vi "inner_product.vi"(8 "L2ENDpos":cluster{"X":sgl, "Y":sgl}={"X"=7.0, "Y"=2.0}, 9 "L2STARTpos":cluster{"X":sgl, "Y":sgl}={"X"=2.0, "Y"=2.0}, 10 "L1ENDpos":cluster{"X":sgl, "Y":sgl}={"X"=1.0, "Y"=1.0}, 11 "L1STARTpos":cluster{"X":sgl, "Y":sgl}={"X"=0.0, "Y"=1.0}) -> (3 "数值":dbl format="%#_13g")   [LabVIEW 2018]
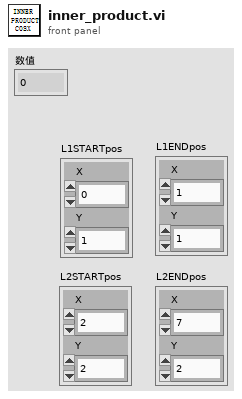
[diagram p1: front panel]
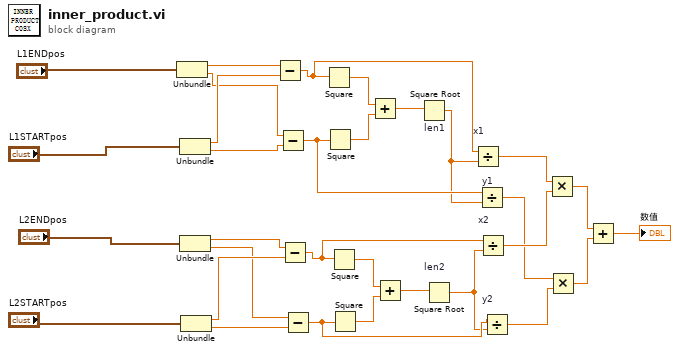
[diagram p0: block diagram]
diagram:
  n1 = Unbundle("L1ENDpos") -> ("X"=w27:sgl, "Y"=w25:sgl)
  n2 = Unbundle("L1STARTpos") -> ("X"=w26:sgl, "Y"=w24:sgl)
  n3 = Unbundle("L2ENDpos") -> ("X"=w17:sgl, "Y"=w15:sgl)
  n4 = Unbundle("L2STARTpos") -> ("X"=w16:sgl, "Y"=w14:sgl)
  n5 = Subtract(x=w27, y=w26) -> (x-y=w13:sgl)
  n6 = Subtract(x=w25, y=w24) -> (x-y=w11:sgl)
  n7 = Subtract(x=w17, y=w16) -> (x-y=w12:sgl)
  n8 = Subtract(x=w15, y=w14) -> (x-y=w9:sgl)
  n9 = Square(x=w13) -> (x^2=w23:sgl)
  n10 = Square(x=w11) -> (x^2=w22:sgl)
  n11 = Square(x=w12) -> (x^2=w20:sgl)
  n12 = Square(x=w9) -> (x^2=w19:sgl)
  n13 = Add(x=w23, y=w22) -> (x+y=w21:sgl)
  n14 = Add(x=w20, y=w19) -> (x+y=w18:sgl)
  n15 = Square Root "len1"(x=w21) -> (sqrt(x)=w10:sgl)
  n16 = Square Root "len2"(x=w18) -> (sqrt(x)=w8:sgl)
  n17 = Divide "x1"(x=w13, y=w10) -> (x/y=w7:sgl)
  n18 = Divide "y1"(x=w11, y=w10) -> (x/y=w5:sgl)
  n19 = Divide "x2"(x=w12, y=w8) -> (x/y=w6:sgl)
  n20 = Divide "y2"(x=w9, y=w8) -> (x/y=w4:sgl)
  n21 = Multiply(x=w7, y=w6) -> (x*y=w2:sgl)
  n22 = Multiply(x=w5, y=w4) -> (x*y=w3:sgl)
  n23 = Add(x=w2, y=w3) -> (x+y=→"数值":sgl)
